vi "DAQNavi Read (Buffered Counter Count Value).vi"(8 "error in (no error)":errorcluster, 9 "number of samples per channel to read":i32=10, 10 "timeout":dbl=10.0, 11 "task in":i32) -> (0 "error out":errorcluster, 2 "data":i32[][](array[numeric]), 3 "task out":i32)   [LabVIEW 2020]
uses:
  DAQNavi_LV.dll
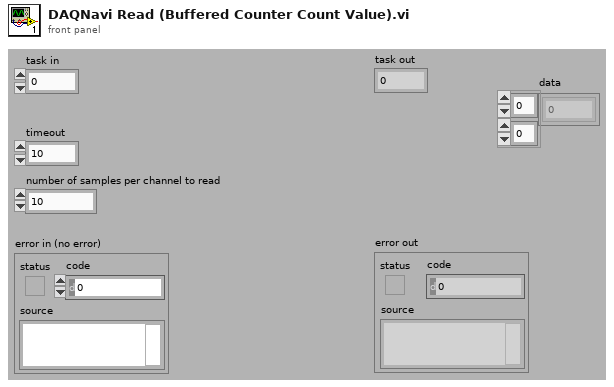
[diagram p1: front panel]
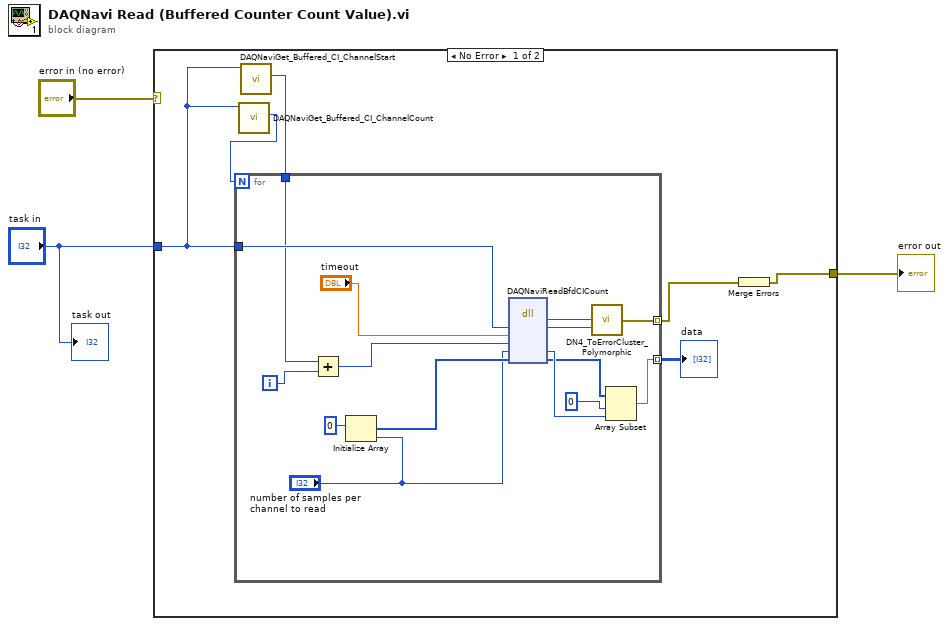
[diagram p0: block diagram]
diagram:
  n1 = case shown="No Error" "error in (no error)" {
    selector: "error in (no error)" -> [_ w25]
    tunnel: "task in" -> [w5 _]
    tunnel: [w7 w25] -> w1
    frame No Error {
      n2 = call "DAQNaviGet_Buffered_CI_ChannelCount.vi"("task in"=w5) -> ("channelCount"=w6:i32)  [unwired: 1 in, 9 out]
      n3 = call "DAQNaviGet_Buffered_CI_ChannelStart.vi"("task in"=w5) -> ("channelStart"=w4:i32)  [unwired: 1 in, 9 out]
      n4 = for {
        N: w6 -> [_]
        tunnel: w5 -> [w24]
        tunnel: [w10] -> w9 mode=indexing
        tunnel: [w16] -> w8 mode=indexing
        tunnel: w4 -> [w15]
        i -> [w19]
        n5 = Add(x=w15, y=w19) -> (x+y=w18:i32)
        n6 = Initialize Array(0, "number of samples per channel to read") -> (w22:i32[])
        n7 = dll-call lib="DAQNavi_LV.dll" fn="DAQNaviReadBfdCICount"("taskID"=w24, "timeout"="timeout", "cntr"=w18, "count"="number of samples per channel to read", "samples"=w22) -> ("return type"=w17:i32, "taskID"=w14:i32, "count"=w13:i32, "samples"=w11:i32[])  [unwired: 5 in, 2 out]
        n8 = call "DN4_ToErrorCluster_Polymorphic.vi"("task id"=w14, "error code"=w17) -> ("error out"=w16:errorcluster)  [unwired: 3 out]
        n9 = Array Subset(array=w11, index=0, length=w13) -> (w10:i32[])
      }
      "data" <- w9
      n10 = Merge Errors(w8) -> (w7:errorcluster)
    }
    frame Error {
    }
  }
  "error out" <- w1
  "task out" <- "task in"
